vi "VNA_agilent_config_freq_sweep.vi"(4 "IF Bandwidth":dbl, 5 "Averaging":i32, 6 "Number of Points":i32, 7 "Output Power":dbl, 8 "error in (no error)":errorcluster, 9 "Stop Frequency":dbl, 10 "Start Frequency":dbl) -> (0 "error out":errorcluster, 3 "Resource Name Out":refnum<k15>)   [LabVIEW 2016]
uses:
  <instrlib>/Keysight PNA Series/Keysight PNA Series.lvlib
panel:
  in  "VISA resource name":refnum<visa-resource-name>
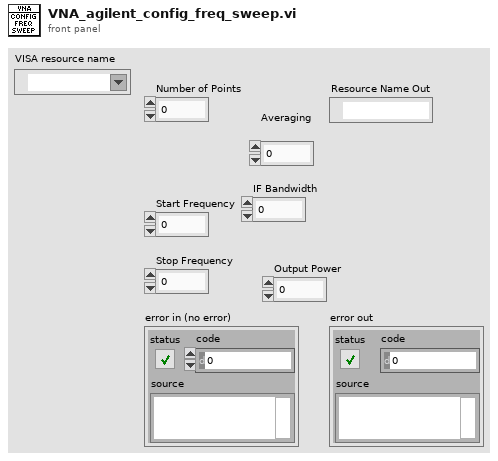
[diagram p1: front panel]
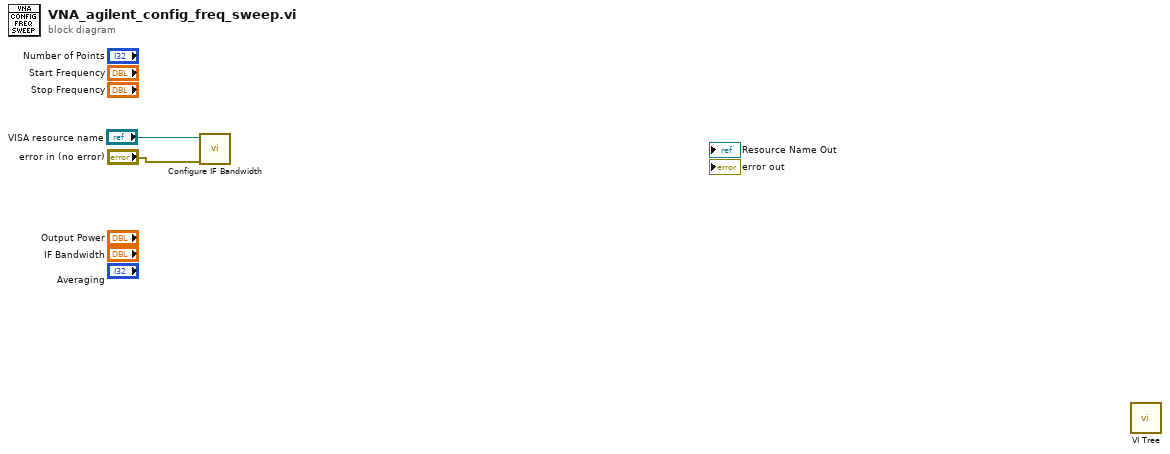
[diagram p0: block diagram]
diagram:
  n1 = call <instrlib>:"Configure IF Bandwidth.vi"("error in (no error)"="error in (no error)", "VISA resource name"="VISA resource name") -> ()  [unwired: 8 in, 2 out]
  n2 = call <instrlib>:"VI Tree.vi"() -> ()  [unwired: 12 in]
